vi "UpdateControls.vi"(6 "50mA Spectra":cluster{"Wavelength":dbl[], "EL Spectrum":dbl[]}, 8 "error in (no error)":errorcluster, 9 "20mA Spectra":cluster{"Wavelength":dbl[], "EL Spectrum":dbl[]}, 10 "Data In":T1 {"50mA Data"."Current,mA" format="%_6g"; "50mA Data"."WL" format="%_6g"; "50mA Data"."Voltage" format="%_6g"; "50mA Data"."Power" format="%_6g"; "20mA Data"."Reverse" format="%#_3g"; "20mA Data"."Current,mA" format="%_6g"; "20mA Data"."Knee Current" format="%#_3g"; "20mA Data"."WL" format="%_6g"; "20mA Data"."Voltage" format="%_6g"; "20mA Data"."Power" format="%_5g"}, 11 "EpiWrapper in":refnum<class "EpiWrapper.lvclass">) -> (0 "error out":errorcluster, 3 "EpiWrapper out":refnum<class "EpiWrapper.lvclass">)   [LabVIEW 2012, in "EpiWrapper.lvclass"]
uses:
  EpiWrapper.lvclass
  Controls/TestData.ctl
  EpiWrapper.lvclass/EpiWrapper.ctl
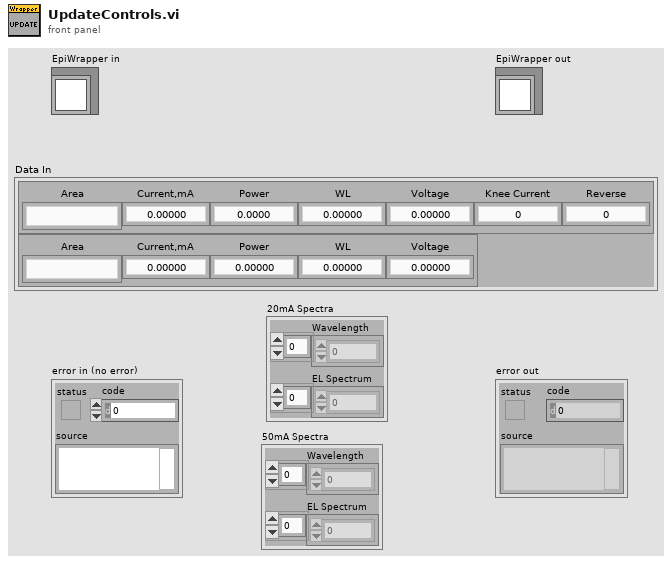
[diagram p1: front panel]
types:
  T1 = typedef "TestData.ctl" = cluster{"20mA Data":cluster{"Area":string, "Current,mA":dbl, "Power":dbl, "WL":dbl, "Voltage":dbl, "Knee Current":dbl, "Reverse":dbl}, "50mA Data":cluster{"Area":string, "Current,mA":dbl, "Power":dbl, "WL":dbl, "Voltage":dbl}}
  T2 = cluster{"Area":string, "Current,mA":dbl, "Power":dbl, "WL":dbl, "Voltage":dbl, "Knee Current":dbl, "Reverse":dbl}
  T3 = typedef "MeasureControl.ctl" = cluster{"Pass":bool, "Fail":bool, "Measure":bool, "Area":T4, "TestData":T1, "Graph":cluster{"Y":dbl[], "Y":dbl[]}[]}
  T4 = typedef "TestArea.ctl" = string
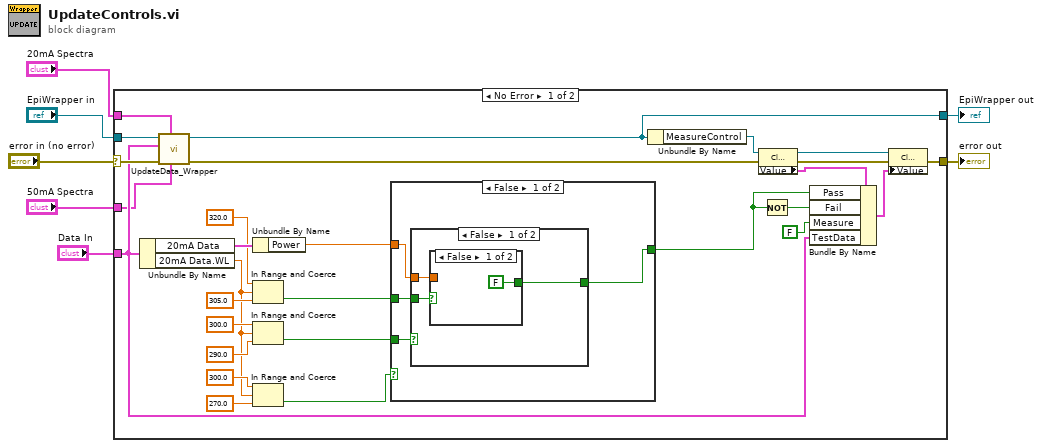
[diagram p0: block diagram]
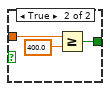
[diagram p2: hidden frame]
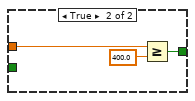
[diagram p3: hidden frame]
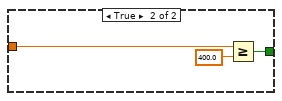
[diagram p4: hidden frame]
diagram:
  n1 = case shown="No Error" "error in (no error)" {
    selector: "error in (no error)" -> [w14 w54]
    tunnel: [w15 w54] -> w6
    tunnel: [w8 w53] -> w4
    tunnel: "EpiWrapper in" -> [w9 w53]
    tunnel: "Data In" -> [w12 _]
    tunnel: "20mA Spectra" -> [w11 _]
    tunnel: "50mA Spectra" -> [w10 _]
    frame No Error {
      n2 = Unbundle By Name(w12) -> ("20mA Data"=w33:T2, "20mA Data.WL"=w19:dbl)
      n3 = call-dynamic "UpdateData_Wrapper.vi"("50mA Spectra"=w10, "20mA Spectra"=w11, "error in (no error)"=w14, "Data In"=w12, "EpiWrapper in"=w9) -> ("error out"=w13:errorcluster, "EpiWrapper out"=w8:refnum<class "EpiWrapper.lvclass">)  [unwired: 5 in]
      n4 = Unbundle By Name(w33) -> ("Power"=w23:dbl)
      n5 = In Range and Coerce(upper limit=320.0, x=w19, lower limit=305.0) -> (In Range?=w24:bool)  [unwired: 1 out]
      n6 = In Range and Coerce(upper limit=300.0, x=w19, lower limit=290.0) -> (In Range?=w25:bool)  [unwired: 1 out]
      n7 = In Range and Coerce(upper limit=300.0, x=w19, lower limit=270.0) -> (In Range?=w26:bool)  [unwired: 1 out]
      n8 = case shown="False" w26 {
        tunnel: w25 -> [w39 _]
        tunnel: w24 -> [w38 _]
        tunnel: w23 -> [w37 w52]
        tunnel: [w36 w50] -> w20
        frame False {
          n9 = case shown="False" w39 {
            tunnel: w38 -> [w42 _]
            tunnel: w37 -> [w41 w48]
            tunnel: [w40 w47] -> w36
            frame False {
              n10 = case shown="False" w42 {
                tunnel: w41 -> [_ w45]
                tunnel: [FALSE w44] -> w40
                frame False {
                }
                frame True {
                  n11 = Greater Or Equal?(x=w45, y=400.0) -> (x >= y?=w44:bool)
                }
              }
            }
            frame True {
              n12 = Greater Or Equal?(x=w48, y=400.0) -> (x >= y?=w47:bool)
            }
          }
        }
        frame True {
          n13 = Greater Or Equal?(x=w52, y=400.0) -> (x >= y?=w50:bool)
        }
      }
      n14 = Unbundle By Name(w8) -> ("MeasureControl"=w35:refnum<vi>)
      n15 = property class="Clust (strict)"(reference=w35, error in=w13) -> (reference out=w17:refnum<vi>, error out=w16:errorcluster, "Value"=w34:T3)
      n16 = Not(x=w20) -> (.not. x?=w22:bool)
      n17 = Bundle By Name(cluster=w34, "Pass"=w20, "Fail"=w22, "Measure"=FALSE, "TestData"=w12) -> (w18:T3)
      n18 = property class="Clust (strict)"(reference=w17, error in=w16, "Value"=w18) -> (error out=w15:errorcluster)  [unwired: 1 out]
    }
    frame Error {
    }
  }
  "error out" <- w6
  "EpiWrapper out" <- w4
